vi "Read.vi"(7 "timeout (100ms)":i32=100, 8 "error in (no error)":errorcluster, 9 "Interlock in":bool, 11 "IL U16 Allow in":refnum<class "IL U16 Pass.lvclass">) -> (0 "error out":errorcluster, 1 "Interlock out":bool, 2 "Data out":variant, 3 "IL U16 Allow out":refnum<class "IL U16 Pass.lvclass">, 4 "IL Action":refnum<class "IL Action.lvclass">[](array[class]))   [LabVIEW 2015, in "Interlocks.lvlib" / "IL U16 Pass.lvclass"]
uses:
  IL U16 Pass.lvclass
  IL Action/IL Action.lvclass
  IL U16 Pass.lvclass/IL U16 Pass.ctl
  Interlock/State Enum.ctl
  Interlock/Interlock.lvclass/Interlock.ctl
  Interlock/Interlock.lvclass
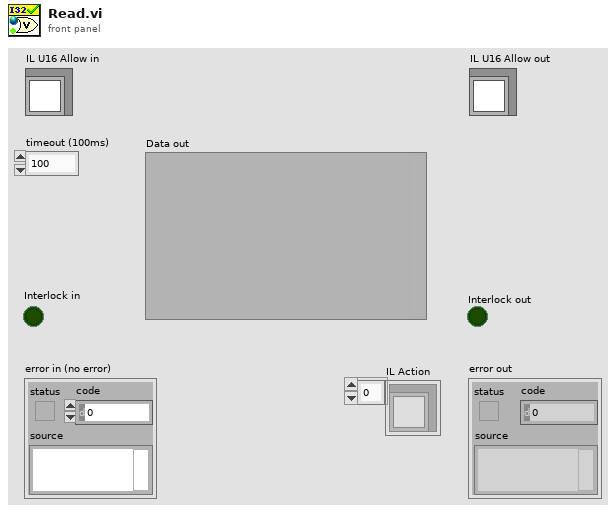
[diagram p1: front panel]
types:
  T1 = typedef "Interlocks.lvlib/Interlock.lvclass/State Enum.ctl" = enum16{"Error", "Ok", "Interlock", "Out of Range", "Is ON", "Is OFF", "Denied", "Not Allowed", "Sample Allow", "Sample Deny"}
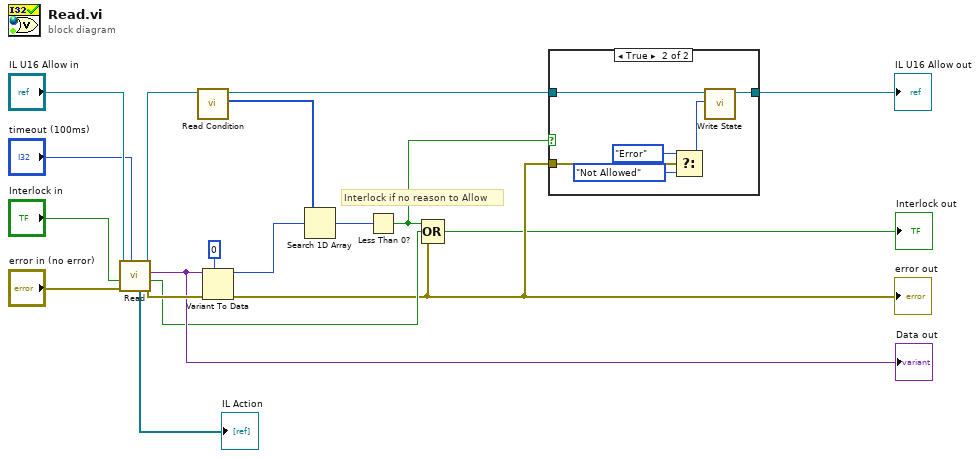
[diagram p0: block diagram]
diagram:
  # "Interlock if no reason to Allow"
  n1 = call-parent "Read.vi"("timeout (100ms)"="timeout (100ms)", "error in (no error)"="error in (no error)", 9:"Interlock in"="Interlock in", 11:"Interlock in"="IL U16 Allow in") -> ("error out"=w15:errorcluster, 1:"Interlock out"=w9:bool, "Data out"=w13:variant, 3:"Interlock out"=w14:refnum<class "IL U16 Pass.lvclass">, "IL Action"=→"IL Action":refnum<class "IL Action.lvclass">[])  [unwired: 3 in]
  "Data out" <- w13
  n2 = call "Read Condition.vi"("IL U16 Allow in"=w14) -> ("Allow"=w12:u16[], "IL U16 Allow out"=w5:refnum<class "IL U16 Pass.lvclass">)  [unwired: 9 in]
  n3 = Variant To Data(error in=w15, type=u16 0, Variant=w13) -> (data=w11:u16, error out=w8:errorcluster)
  "error out" <- w8
  n4 = Search 1D Array(1D array=w12, element=w11) -> (index of element=w10:i32)  [unwired: 1 in]
  n5 = Less Than 0?(x=w10) -> (x < 0?=w6:bool)
  n6 = Compound Arithmetic op=OR(w6, w9, w8) -> (→"Interlock out":bool)
  n7 = case shown="True" w6 {
    tunnel: w8 -> [_ w25]
    tunnel: w5 -> [w19 w22]
    tunnel: [w19 w21] -> w4
    frame False {
    }
    frame True {
      n8 = Select(t=State_Enum."Error", s=w25, f=State_Enum."Not Allowed" ("State")) -> (s? t:f=w20:T1)
      n9 = call "Write State.vi"("State"=w20, "Interlock in"=w22) -> ("Interlock out"=w21:refnum<class "IL U16 Pass.lvclass">)  [unwired: 9 in]
    }
  }
  "IL U16 Allow out" <- w4
